vi "UTIL Read CSV.vi"(1 "CSV Path":path) -> (0 "Data From File":dbl[][](array[numeric]))   [LabVIEW 2017]
doc: "Read data from a CSV file.\n\nInput\n CSV Path Path Constant\nOutput \n Data from File 2-D Array of DBL"
uses:
  <vilib>/Utility/file.llb/Read Delimited Spreadsheet (DBL).vi
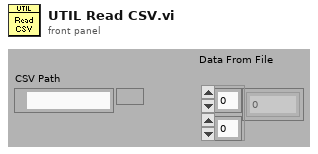
[diagram p1: front panel]
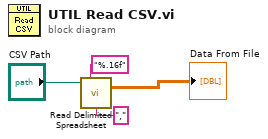
[diagram p0: block diagram]
diagram:
  n1 = call-poly <vilib>:"Read Delimited Spreadsheet.vi"("file path (dialog if empty)"="CSV Path", "format (%.3f)"="%.16f", "delimiter (\\t)"="," ("delimiter (\\t)")) -> ("all rows"=→"Data From File":dbl[][])  [unwired: 7 in, 5 out]
